vi "Debug Dequeuer.vi"() -> ()   [LabVIEW 2013]
panel:
  out "Z Waveform Chart":waveform(dbl)[](graph)
  out "Y Waveform Chart":waveform(dbl)[](graph)
  out "X Waveform Chart":waveform(dbl)[](graph)
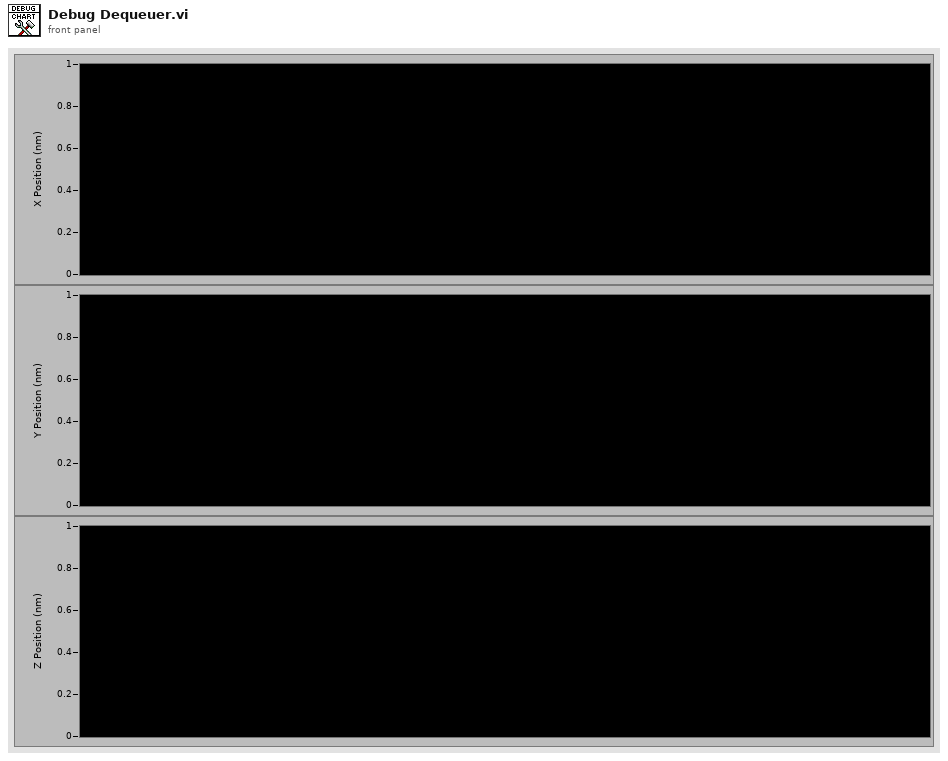
[diagram p1: front panel]
types:
  T1 = typedef "Debug Queue.ctl" = refnum<queue>
  T2 = typedef "Experimental Configuration.ctl" = cluster{"Output Waveforms":waveform(dbl)[], "Output Channels":string, "Input Channels":string, "Post-Hook Occurence":refnum<k4>}
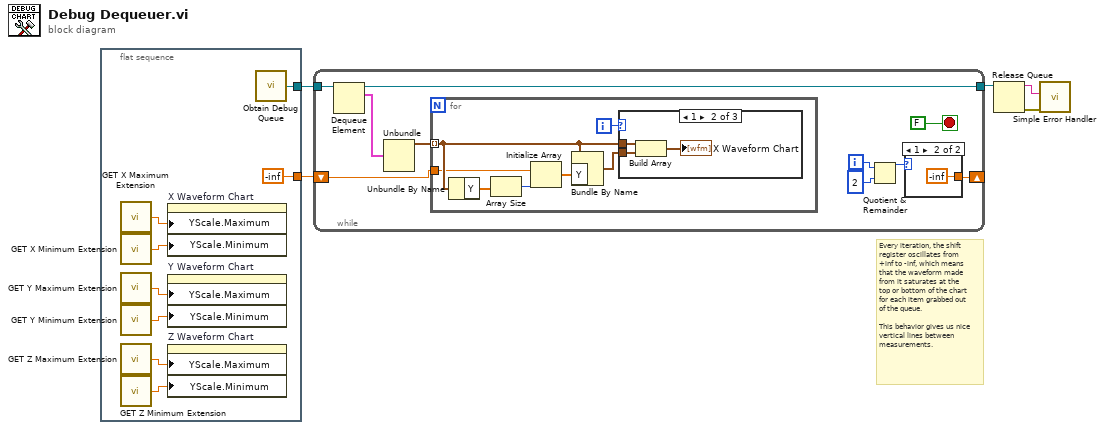
[diagram p0: block diagram]
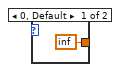
[diagram p2: hidden frame]
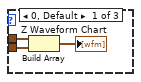
[diagram p3: hidden frame]
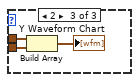
[diagram p4: hidden frame]
diagram:
  # "Every iteration, the shift\nregister oscillates from\n+inf to -inf, which means\nthat the waveform made\nfrom it saturates at the\ntop or bottom of the chart\nfor each item grabbed out\nof the queue.\n\nThis behavior gives us nice\nvertical lines between\nmeasurements."
  n1 = flat-sequence {
    tunnel: [w13] -> w5
    tunnel: [-inf] -> w1
    frame #0 {
      n2 = call "GET X Maximum Extension.vi"() -> ("X Maximum Extension"=w12:dbl)
      n3 = call "GET X Minimum Extension.vi"() -> ("X Minimum Extension"=w11:dbl)
      n4 = call "GET Y Maximum Extension.vi"() -> ("Y Maximum Extension"=w10:dbl)
      n5 = call "GET Y Minimum Extension.vi"() -> ("Y Minimum Extension"=w9:dbl)
      n6 = call "GET Z Maximum Extension.vi"() -> ("Z Maximum Extension"=w8:dbl)
      n7 = call "GET Z Minimum Extension.vi"() -> ("Z Minimum Extension"=w7:dbl)
      n8 = property on="X Waveform Chart" class="WFChart (strict)"("YScale.Maximum"=w12, "YScale.Minimum"=w11) -> ()  [unwired: 2 in, 2 out]
      n9 = property on="Y Waveform Chart" class="WFChart (strict)"("YScale.Maximum"=w10, "YScale.Minimum"=w9) -> ()  [unwired: 2 in, 2 out]
      n10 = property on="Z Waveform Chart" class="WFChart (strict)"("YScale.Maximum"=w8, "YScale.Minimum"=w7) -> ()  [unwired: 2 in, 2 out]
      n11 = call "Obtain Debug Queue.vi"() -> ("Debug Queue"=w13:T1)
    }
  }
  n12 = while {
    tunnel: w5 -> [w22]
    tunnel: [w21] -> w4
    shift-right: [w15] -> _
    shift-left: w1 -> [w14]
    i -> [w18]
    stop <- FALSE stop-if-true
    n13 = Dequeue Element(queue=w22) -> (queue out=w21:T1, element=w20:T2)  [unwired: 2 in, 2 out]
    n14 = Unbundle(w20) -> ("Output Waveforms"=w19:waveform(dbl)[])  [unwired: 3 out]
    n15 = for {
      tunnel: w19 -> [w30] mode=indexing
      tunnel: w14 -> [w26]
      i -> [w32]
      n16 = Unbundle By Name(w30) -> ("Y"=w29:dbl[])
      n17 = Array Size(array=w29) -> (size(s)=w28:i32)
      n18 = Initialize Array(w26, w28) -> (w27:dbl[])
      n19 = Bundle By Name(cluster=w30, "Y"=w27) -> (w31:waveform(dbl))
      n20 = case shown="1" w32 {
        tunnel: w30 -> [w35 w38 w41]
        tunnel: w31 -> [w33 w36 w39]
        frame 0, Default {
          n21 = Build Array(w35, w33) -> (→"Z Waveform Chart":waveform(dbl)[])
        }
        frame 1 {
          n22 = Build Array(w38, w36) -> (→"X Waveform Chart":waveform(dbl)[])
        }
        frame 2 {
          n23 = Build Array(w41, w39) -> (→"Y Waveform Chart":waveform(dbl)[])
        }
      }
    }
    n24 = Quotient & Remainder(x=w18, y=2) -> (x-y*floor(x/y)=w16:i32)  [unwired: 1 out]
    n25 = case shown="1" w16 {
      tunnel: [inf -inf] -> w15
      frame 0, Default {
      }
      frame 1 {
      }
    }
  }
  n26 = Release Queue(queue=w4) -> (queue name=w3:string, error out=w2:errorcluster)  [unwired: 2 in, 1 out]
  n27 = call <vilib>:"Simple Error Handler.vi"("error source (\" \")"=w3, "error in (no error)"=w2) -> ()  [unwired: 3 in, 5 out]
